vi "Stop Core.vi"(10 "final error code":i32, 11 "AssertEngine in":refnum<class "AssertEngine.lvclass">) -> (3 "AssertEngine out":refnum<class "AssertEngine.lvclass">)   [LabVIEW 2016, in "AssertEngine.lvlib" / "AssertEngine.lvclass"]
doc: "(<B>Filename</B>: Actor Framework.lvlib:Actor.lvclass:Stop Core.vi)\n\nDefines what the actor does before it stops. Use the <B>final error code</B> input to determine whether the actor shut down in response to an error.\n\nBy default, this method does nothing. A descendant class may override it to define behavior, such as shutting down any processes the actor initiated in its override of the Actor Core method."
uses:
  AssertEngine.lvclass
  External Message Queue/Classes/Stop/Stop Helper.lvclass
  D:/Work/Projects/Actor_Assert_API/AssertEngine/External Message Queue/Classes/External Msg.lvclass
  AssertEngine.lvclass/AssertEngine.ctl
  <vilib>/ActorFramework/Message Enqueuer/Message Enqueuer.lvclass/Message Enqueuer.ctl
  <vilib>/ActorFramework/Message Enqueuer/Enqueue.vi
  <vilib>/ActorFramework/Stop Msg/Stop Msg.lvclass
  C:/Program Files/National Instruments/LabVIEW 2016/vi.lib/ActorFramework/Message/Message.lvclass
  <vilib>/ActorFramework/Message Priority Queue/Priority Enqueue.vi
  <vilib>/ActorFramework/Actor/Actor.lvclass
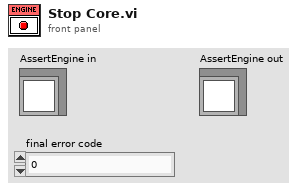
[diagram p1: front panel]
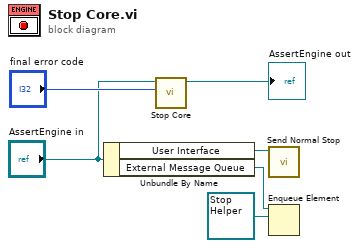
[diagram p0: block diagram]
diagram:
  n1 = Unbundle By Name("AssertEngine in") -> ("User Interface"=w3:refnum<class "Message Enqueuer.lvclass">, "External Message Queue"=w2:refnum<queue>)
  n2 = call-parent "Stop Core.vi"("final error code"="final error code", "Actor in"="AssertEngine in") -> ("Actor out"=→"AssertEngine out":refnum<class "AssertEngine.lvclass">)  [unwired: 9 in]
  n3 = call <vilib>:"Send Normal Stop.vi"("Message Enqueuer"=w3) -> ()  [unwired: 10 in, 1 out]
  n4 = Enqueue Element(queue=w2, element=refnum<class "Stop Helper.lvclass"> refnum ("AssertEngine.lvlib:Stop Helper.lvclass")) -> ()  [unwired: 2 in, 3 out]
